vi "lab2SwapChannels.vi"(0 "redChannel in":u8[](array[numeric]), 1 "greenChannel in":u8[](array[numeric]), 2 "blueChannel in":u8[](array[numeric]), 3 "swapRg":bool, 4 "swapRb":bool, 5 "swapGb":bool, 7 "bypass":bool) -> (14 "redChannel out":u8[](array[numeric]), 15 "greenChannel out":u8[](array[numeric]), 16 "blueChannel out":u8[](array[numeric]))   [LabVIEW 2016]
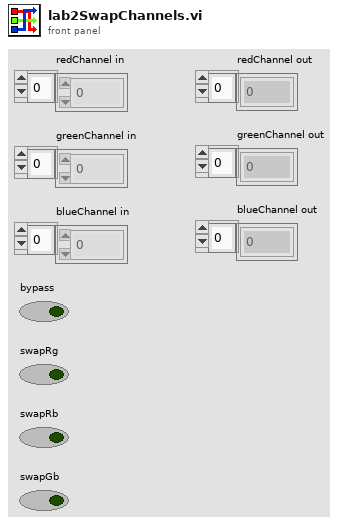
[diagram p1: front panel]
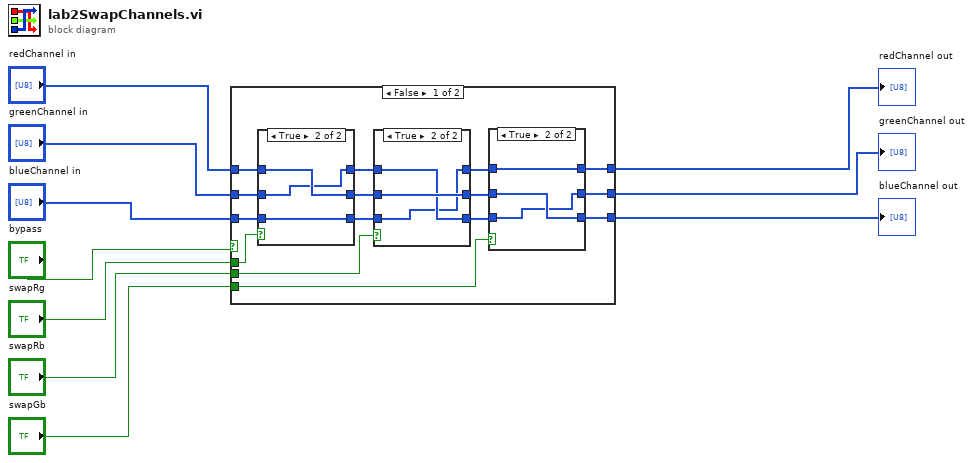
[diagram p0: block diagram]
diagram:
  n1 = case shown="False" "bypass" {
    tunnel: "redChannel in" -> [w19 w46]
    tunnel: "greenChannel in" -> [w18 w45]
    tunnel: "blueChannel in" -> [w17 w44]
    tunnel: [w16 w46] -> w5
    tunnel: [w15 w45] -> w6
    tunnel: [w14 w44] -> w7
    tunnel: "swapRg" -> [w13 _]
    tunnel: "swapRb" -> [w12 _]
    tunnel: "swapGb" -> [w11 _]
    frame False {
      n2 = case shown="True" w13 {
        tunnel: w17 -> [w40 w41]
        tunnel: w18 -> [w39 w42]
        tunnel: w19 -> [w38 w43]
        tunnel: [w40 w41] -> w22
        tunnel: [w39 w43] -> w23
        tunnel: [w38 w42] -> w25
        frame False {
        }
        frame True {
        }
      }
      n3 = case shown="True" w12 {
        tunnel: w22 -> [w34 w35]
        tunnel: w23 -> [w33 w37]
        tunnel: w25 -> [w32 w36]
        tunnel: [w34 w36] -> w20
        tunnel: [w33 w37] -> w21
        tunnel: [w32 w35] -> w24
        frame False {
        }
        frame True {
        }
      }
      n4 = case shown="True" w11 {
        tunnel: w20 -> [w28 w29]
        tunnel: w21 -> [w27 w30]
        tunnel: w24 -> [w26 w31]
        tunnel: [w28 w30] -> w14
        tunnel: [w27 w29] -> w15
        tunnel: [w26 w31] -> w16
        frame False {
        }
        frame True {
        }
      }
    }
    frame True {
    }
  }
  "blueChannel out" <- w7
  "greenChannel out" <- w6
  "redChannel out" <- w5
